vi "Read Trigger Level.vi"(8 "error in (no error)":errorcluster, 11 "T560Trigger in":refnum<class "T560Trigger.lvclass">) -> (0 "error out":errorcluster, 2 "Trigger Level":string, 3 "T560Trigger out":refnum<class "T560Trigger.lvclass">)   [LabVIEW 2013, in "T560Trigger.lvclass"]
uses:
  T560Trigger.lvclass
  T560Trigger.lvclass/T560Trigger.ctl
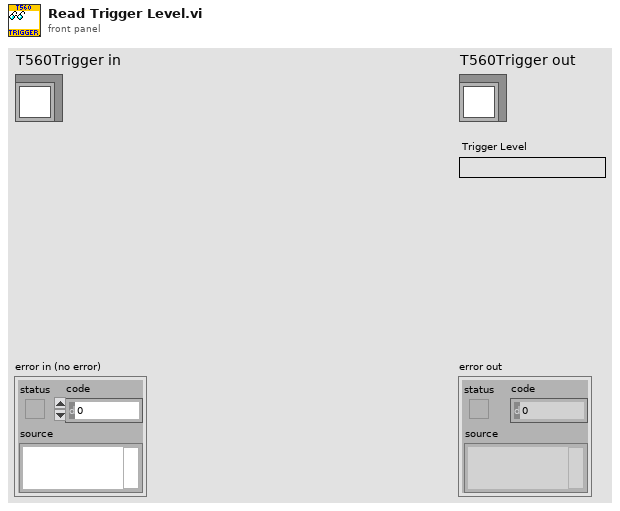
[diagram p1: front panel]
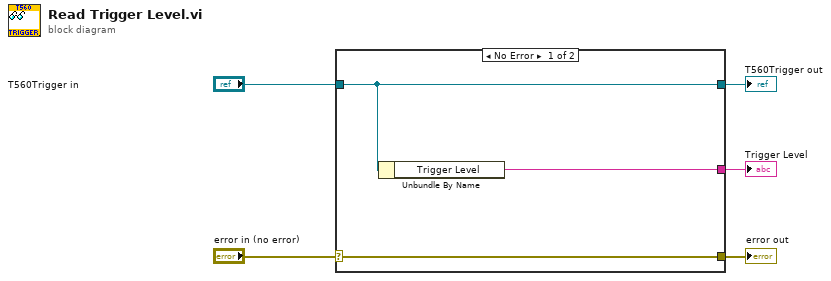
[diagram p0: block diagram]
diagram:
  n1 = case shown="No Error" "error in (no error)" {
    selector: "error in (no error)" -> [w8 w9]
    tunnel: [w8 w9] -> w4
    tunnel: [w7 w10] -> w2
    tunnel: "T560Trigger in" -> [w7 w10]
    tunnel: [w6 _] -> w1
    frame No Error {
      n2 = Unbundle By Name(w7) -> ("Trigger Level"=w6:string)
    }
    frame Error {
    }
  }
  "error out" <- w4
  "T560Trigger out" <- w2
  "Trigger Level" <- w1
